vi "Live_data_feed.vi"() -> ()   [LabVIEW 2016]
panel:
  in  "stop 2":bool
  in  "STOP ALL 2":bool
  out "element":dbl[](array[numeric])
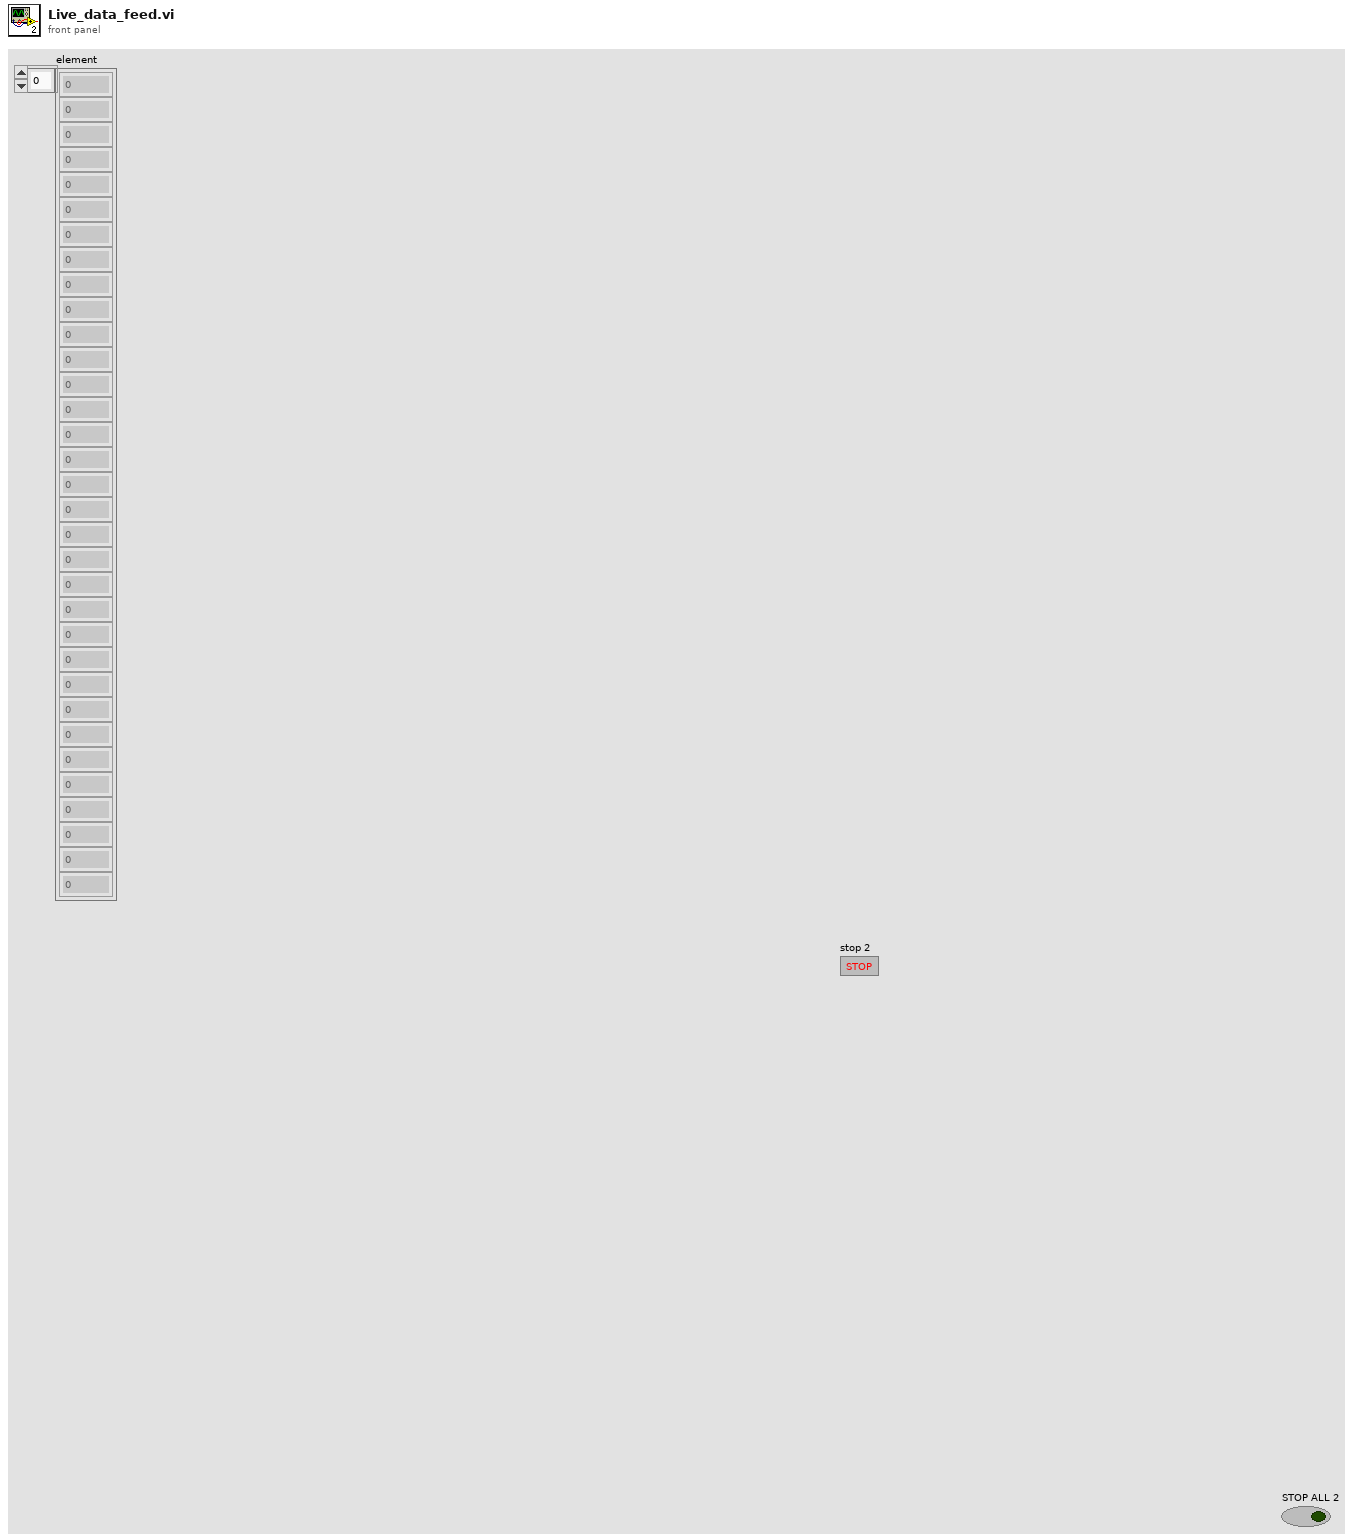
[diagram p1: front panel]
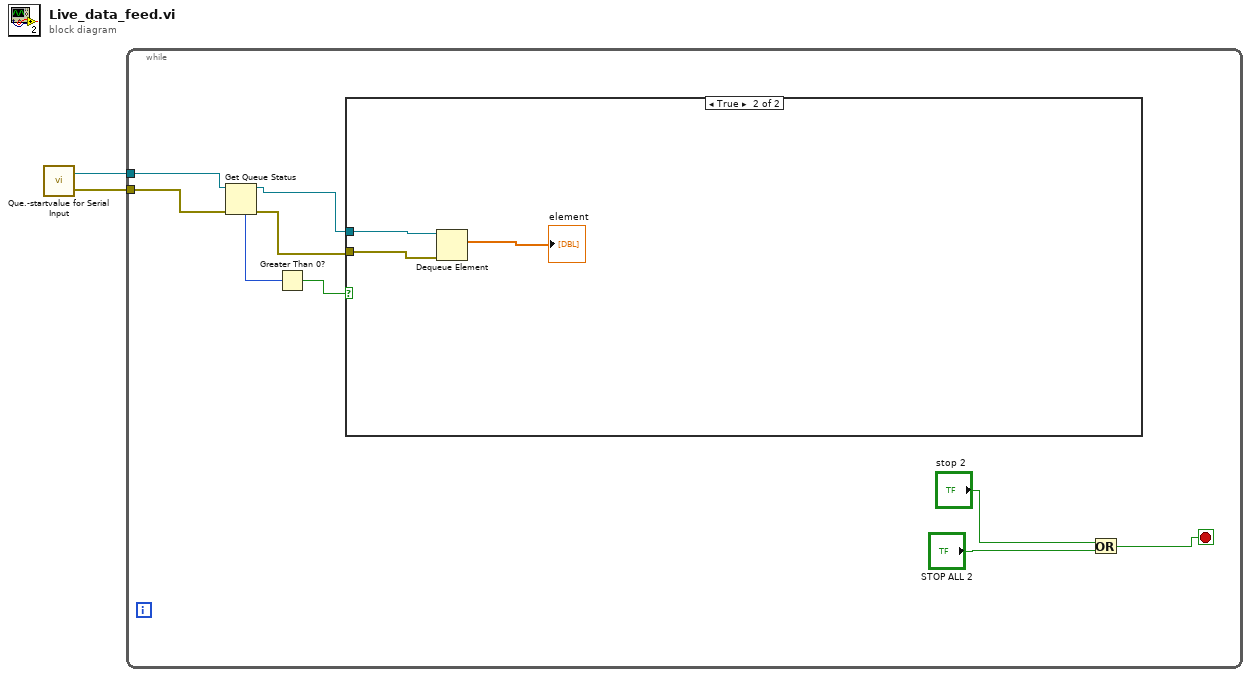
[diagram p0: block diagram]
diagram:
  n1 = call "Que.-startvalue for Serial Input.vi"() -> ("error out"=w1:errorcluster, "queue out"=w2:refnum<queue>)  [unwired: 2 in]
  n2 = while {
    tunnel: w2 -> [w11]
    tunnel: w1 -> [w10]
    stop <- w4 stop-if-true
    n3 = Get Queue Status(queue=w11, error in (no error)=w10) -> (queue out=w7:refnum<queue>, error out=w8:errorcluster, # elements in queue=w6:i32)  [unwired: 1 in, 5 out]
    n4 = Greater Than 0?(x=w6) -> (x > 0?=w9:bool)
    n5 = case shown="True" w9 {
      tunnel: w8 -> [_ w14]
      tunnel: w7 -> [_ w13]
      frame False {
      }
      frame True {
        n6 = Dequeue Element(queue=w13, error in (no error)=w14) -> (element=→"element":dbl[])  [unwired: 1 in, 3 out]
      }
    }
    n7 = Or(x="stop 2", y="STOP ALL 2") -> (x .or. y?=w4:bool)
  }
